vi "Credit Update Coins.vi"(8 "error in (no error)":errorcluster, 10 "Credito":dbl, 11 "UI Actor in":refnum<class "UI Actor.lvclass">) -> (0 "error out":errorcluster, 3 "UI Actor out":refnum<class "UI Actor.lvclass">)   [LabVIEW 2019, in "UI Actor.lvlib" / "UI Actor.lvclass"]
uses:
  UI Actor.lvclass
  UI Actor.lvclass/UI Actor.ctl
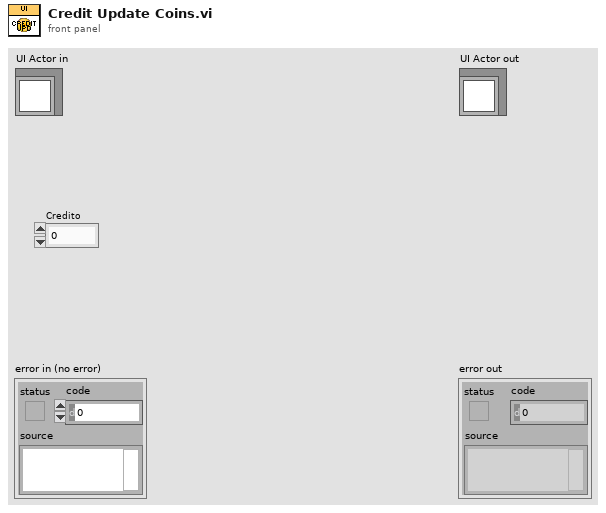
[diagram p1: front panel]
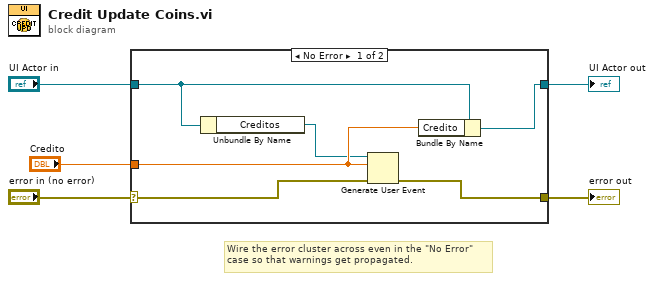
[diagram p0: block diagram]
diagram:
  # "Wire the error cluster across even in the \"No Error\"\ncase so that warnings get propagated."
  n1 = case shown="No Error" "error in (no error)" {
    selector: "error in (no error)" -> [w11 w13]
    tunnel: [w10 w13] -> w4
    tunnel: [w8 w12] -> w2
    tunnel: "UI Actor in" -> [w9 w12]
    tunnel: "Credito" -> [w7 _]
    frame No Error {
      n2 = Unbundle By Name(w9) -> ("Creditos"=w6:refnum<user-event>)
      n3 = Generate User Event(user event=w6, event data cluster=w7, error in=w11) -> (error out=w10:errorcluster)  [unwired: 1 in, 1 out]
      n4 = Bundle By Name(cluster=w9, "Credito"=w7) -> (w8:refnum<class "UI Actor.lvclass">)
    }
    frame Error {
    }
  }
  "error out" <- w4
  "UI Actor out" <- w2
